vi "Chroma_19020_AC&IR_Set.vi"(8 "error in (no error)":errorcluster caption="错误输入（无错误）", 11 "configuration file path":path) -> (0 "error out":errorcluster caption="错误输出")   [LabVIEW 2018]
uses:
  Subvi/Global.vi
  <vilib>/Instr/_visa.llb/VISA Configure Serial Port (Instr).vi
panel:
  out "IR CMD":string[](array[string])
  out "AC CMD":string[](array[string])
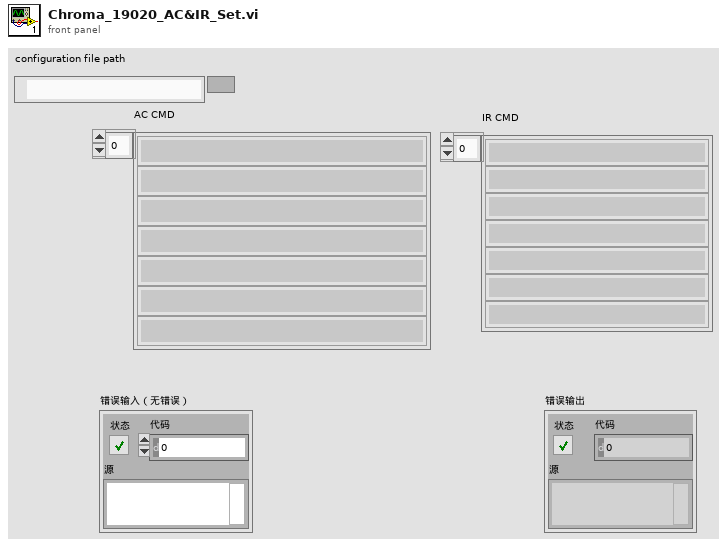
[diagram p1: front panel]
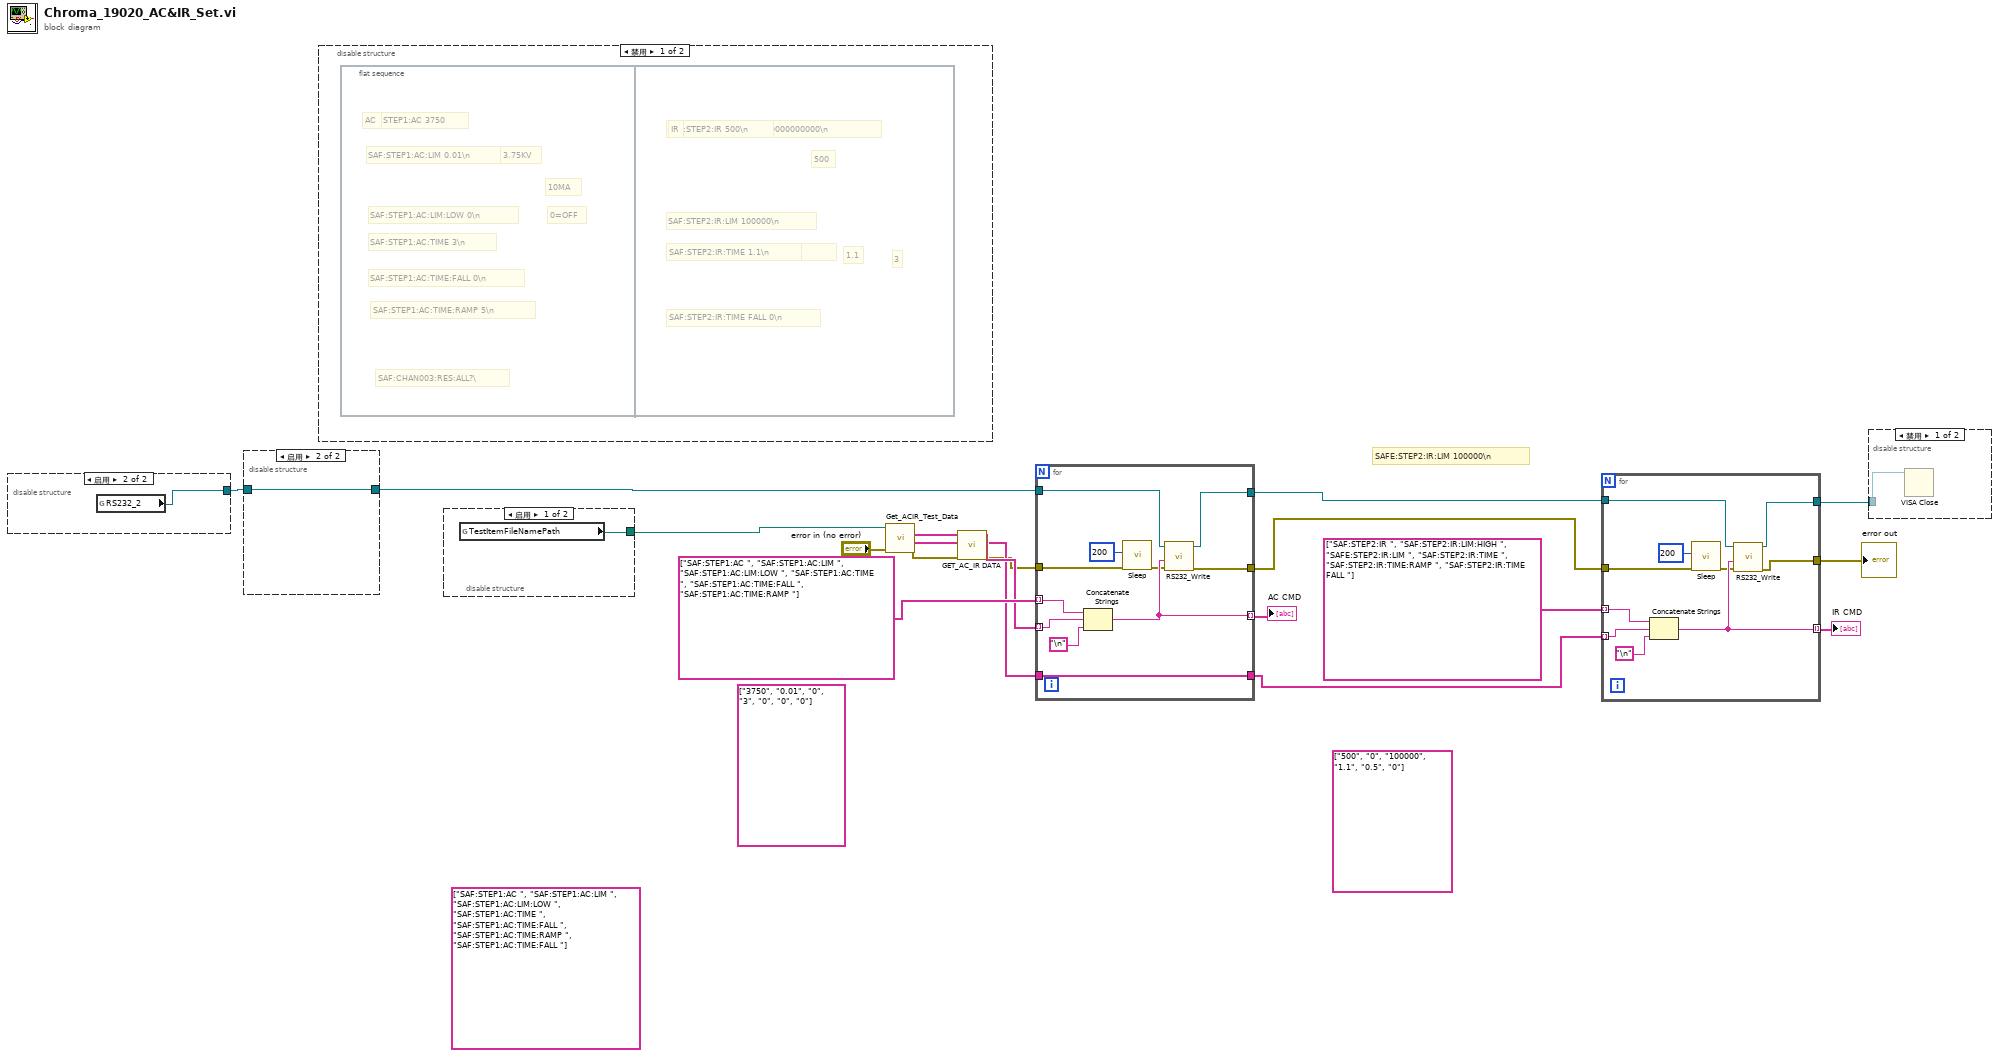
[diagram p0: block diagram]
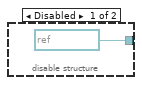
[diagram p2: hidden frame]
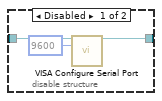
[diagram p4: hidden frame]
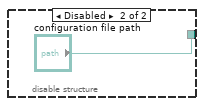
[diagram p5: hidden frame]
diagram:
  (unwired) string[] ["500", "0", "100000", "1.1", "0.5", "0"]
  (unwired) string[] ["3750", "0.01", "0", "3", "0", "0", "0"]
  (unwired) string[] ["SAF:STEP1:AC ", "SAF:STEP1:AC:LIM ", "SAF:STEP1:AC:LIM:LOW ", "SAF:STEP1:AC:TIME ", "SAF:STEP1:AC:TIME:FALL ", "SAF:STEP1:AC:TIME:RAMP ", "SAF:STEP1:AC:TIME:FALL "]
  # "SAFE:STEP2:IR:LIM 100000\\n"
  n1 = disable-structure shown="启用" {
    disable-tunnel: [refnum<visa-resource-name> "COM4" ("VISA资源名称") w21] -> w19
    frame Disabled {
    }
    frame Enabled {
      n2 = global read "Global.vi" "RS232_2"() -> (w21:refnum<visa-resource-name>)
    }
  }
  n3 = disable-structure shown="启用" {
    disable-tunnel: w19 -> [w24 w25]
    disable-tunnel: [w23 w25] -> w9
    frame Disabled {
      n4 = call-poly "VISA Configure Serial Port"("VISA resource name"=w24, "baud rate (9600)"=u32 9600) -> ("VISA resource name out"=w23:refnum<visa-resource-name>)  [unwired: 12 in, 1 out]
    }
    frame Enabled {
    }
  }
  n5 = disable-structure shown="禁用" {
    frame Disabled {
      n6 = flat-sequence {
        frame #0 {
          # "SAF:CHAN003:RES:ALL?\\"
          # "AC"
          # "SAF:STEP1:AC:TIME:RAMP 5\\n"
          # "SAF:STEP1:AC:TIME:FALL 0\\n"
          # "SAF:STEP1:AC:TIME 3\\n"
          # "0=OFF"
          # "SAF:STEP1:AC:LIM:LOW 0\\n"
          # "10MA"
          # "3.75KV"
          # "SAF:STEP1:AC:LIM 0.01\\n"
          # "SAF:STEP1:AC:TIME:FALL 0\\n"
          # "SAF:STEP1:AC 3750"
        }
        frame #1 {
          # "3"
          # "1.1"
          # "500"
          # "IR"
          # "SAF:STEP2:IR:TIME 1.1\\n"
          # "SAF:STEP2:IR:TIME FALL 0\\n"
          # "SAF:STEP2:IR:TIME:RAMP 0.5\\n"
          # "SAF:STEP2:IR:LIM:HIGH 50000000000\\n"
          # "SAF:STEP2:IR:LIM 100000\\n"
          # "SAF:STEP2:IR 500\\n"
        }
      }
    }
    frame Enabled {
    }
  }
  n7 = disable-structure shown="启用" {
    disable-tunnel: [w26 "configuration file path"] -> w14
    frame Enabled {
      n8 = global read "Global.vi" "TestItemFileNamePath"() -> (w26:path)
    }
    frame Disabled {
    }
  }
  n9 = call "Get_ACIR_Test_Data.vi"("error in (no error)"="error in (no error)", "configuration file path"=w14) -> ("error out"=w2:errorcluster, "IR_SET DATA"=w4:string[], "AC_SET DATA"=w6:string[])  [unwired: 7 in]
  n10 = call "GET_AC_IR DATA.vi"("error in (no error)"=w2, "IR_SET DATA"=w4, "AC_SET DATA"=w6) -> ("error out"=w1:errorcluster, "IR SET DATA OUT"=w3:string[], "AC SET DATA OUT"=w5:string[])  [unwired: 6 in]
  n11 = for {
    tunnel: w9 -> [w38]
    tunnel: string[] ["SAF:STEP1:AC ", "SAF:STEP1:AC:LIM ", "SAF:STEP1:AC:LIM:LOW ", "SAF:STEP1:AC:TIME ", "SAF:STEP1:AC:TIME:FALL ", "SAF:STEP1:AC:TIME:RAMP "] -> [w37] mode=indexing
    tunnel: w5 -> [w36] mode=indexing
    tunnel: [w34] -> w18
    tunnel: [w33] -> w16 mode=indexing
    tunnel: w1 -> [w32]
    tunnel: w3 -> [w31]
    tunnel: [w31] -> w13
    tunnel: [w30] -> w10
    n12 = Concatenate Strings(w37, w36, "\n") -> (w33:string)
    n13 = call "Sleep.vi"("error in (no error)"=w32, "等待时间（毫秒）"=u32 200) -> ("error out"=w29:errorcluster)  [unwired: 9 in]
    n14 = call "RS232_Write.vi"("错误输入（无错误）"=w29, "写入缓冲区"=w33, "VISA资源名称"=w38) -> ("错误输出"=w30:errorcluster, "VISA资源名称输出"=w34:refnum<visa-resource-name>)  [unwired: 7 in]
  }
  "AC CMD" <- w16
  n15 = for {
    tunnel: w18 -> [w48]
    tunnel: string[] ["SAF:STEP2:IR ", "SAF:STEP2:IR:LIM:HIGH ", "SAFE:STEP2:IR:LIM ", "SAF:STEP2:IR:TIME ", "SAF:STEP2:IR:TIME:RAMP ", "SAF:STEP2:IR:TIME FALL "] -> [w47] mode=indexing
    tunnel: w13 -> [w46] mode=indexing
    tunnel: [w44] -> w8
    tunnel: [w43] -> w15 mode=indexing
    tunnel: [w42] -> w11
    tunnel: w10 -> [w41]
    n16 = Concatenate Strings(w47, w46, "\n") -> (w43:string)
    n17 = call "Sleep.vi"("error in (no error)"=w41, "等待时间（毫秒）"=u32 200) -> ("error out"=w40:errorcluster)  [unwired: 9 in]
    n18 = call "RS232_Write.vi"("错误输入（无错误）"=w40, "写入缓冲区"=w43, "VISA资源名称"=w48) -> ("错误输出"=w42:errorcluster, "VISA资源名称输出"=w44:refnum<visa-resource-name>)  [unwired: 7 in]
  }
  "IR CMD" <- w15
  "error out" <- w11
  n19 = disable-structure shown="禁用" {
    disable-tunnel: w8 -> [w49 _]
    frame Disabled {
      n20 = VISA Close(VISA resource name=w49) -> ()  [unwired: 1 in, 1 out]
    }
    frame Enabled {
    }
  }
